vi "buildWithGCLI.vi"   [LabVIEW 2019, in "Build.lvlib"]
doc: "Use the command line to call this method. See block diagram for command syntax."
uses:
  Build.lvlib
  <vilib>/Wiresmith Technology/G CLI/CLI Class/CLI.lvclass
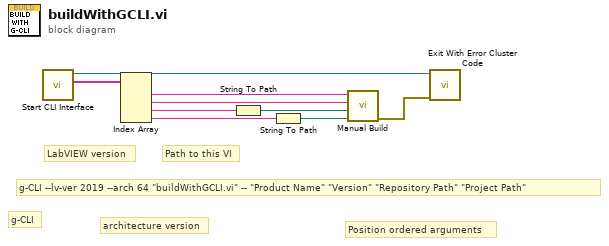
[diagram p0: block diagram]
diagram:
  # "Position ordered arguments"
  # "Path to this VI"
  # "architecture version"
  # "LabVIEW version"
  # "g-CLI"
  # "g-CLI --lv-ver 2019 --arch 64 \"buildWithGCLI.vi\" -- \"Product Name\" \"Version\" \"Repository Path\" \"Project Path\""
  n1 = call <vilib>:"Start CLI Interface.vi"() -> ("Custom Parameters"=w9:string[], "CLI out"=w8:refnum<class "CLI.lvclass">)  [unwired: 8 in, 2 out]
  n2 = Index Array(array=w9) -> (element #1=w6:string, element #2=w5:string, element #3=w4:string, element #4=w3:string)  [unwired: 4 in]
  n3 = String To Path(string=w4) -> (path=w2:path)
  n4 = String To Path(string=w3) -> (path=w1:path)
  n5 = call "Manual Build.vi"("Path to project"=w1, "Path to repository"=w2, "Package Version"=w5, "Product Name"=w6) -> ("Error Out"=w7:errorcluster)  [unwired: 7 in]
  n6 = call <vilib>:"Exit With Error Cluster Code.vi"("error in (no error)"=w7, "CLI in"=w8) -> ()  [unwired: 9 in, 1 out]
